vi "UV-VIS CoolerON.vi"(3 "error in (no error)":errorcluster, 5 "UV-VIS  in":refnum<class "UV-VIS.lvclass">) -> (0 "error out":errorcluster, 1 "DLL error code":u32, 2 "UV-VIS  out":refnum<class "UV-VIS.lvclass">)   [LabVIEW 2015, in "UV-VIS.lvclass"]
doc: "Switches ON the cooling. The rate of temperature change is controlled until the temperature is within 3 degrees of the set value. Control is returned immediately to the calling application.\n\n<B>Error codes:</B>\nDRV_SUCCESS - Temperature controller switched ON.\nDRV_NOT_INITIALIZED - System not initialized.\nDRV_ACQUIRING - Acquisition in progress.\nDRV_ERROR_ACK - Unable to communicate with card.\n\n<B>NOTES:</B>\n<B>The temperature to which the detector will be cooled is set via SetTemperature. The temperature stabilization is controlled via hardware, but the current temperature can be obtained via GetTemperature. The temperature of the sensor is gradually brought to the desired temperature to ensure no thermal stresses are set up in the sensor.</B>"
uses:
  UV-VIS.lvclass
  Detector.lvclass/Detector.ctl
  Detector.lvclass
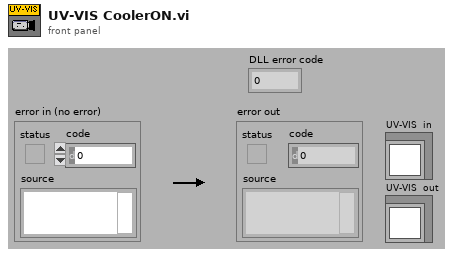
[diagram p1: front panel]
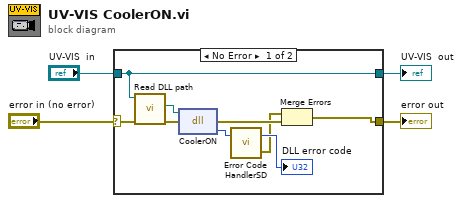
[diagram p0: block diagram]
diagram:
  n1 = case shown="No Error" "error in (no error)" {
    selector: "error in (no error)" -> [w9 w15]
    tunnel: [w5 w15] -> w3
    tunnel: [w8 w14] -> w2
    tunnel: "UV-VIS  in" -> [w8 w14]
    frame No Error {
      n2 = call "Read DLL path.vi"("error in (no error)"=w9, "Detector in"=w8) -> ("error out"=w6:errorcluster, "DLL path"=w7:path)  [unwired: 7 in, 1 out]
      n3 = dll-call lib="S:/TRANCON/DLL/Atmcd32d.dll" fn="CoolerON"(path in=w7, error in=w6) -> (error out=w11:errorcluster, "return type"=w13:u32)  [unwired: 1 in, 1 out]
      n4 = call "Error Code HandlerSD.vi"("DLL error code"=w13) -> ("error out"=w10:errorcluster, "dup DLL error code"=→"DLL error code":u32)  [unwired: 1 in]
      n5 = Merge Errors(w10, w11) -> (w5:errorcluster)
    }
    frame Error {
    }
  }
  "error out" <- w3
  "UV-VIS  out" <- w2
